vi "WheeChromGlobals.vi"() -> ()   [LabVIEW 2020]
panel:
  in  "WavelengthCal":dbl[](array[numeric])
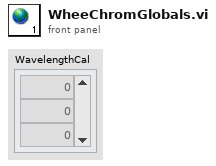
[diagram p1: front panel]
diagram:
